vi "State Exit.vi"(8 "error in":errorcluster, 11 "Context in":refnum<class "State Pattern.lvclass">) -> (0 "error out":errorcluster, 3 "Context out":refnum<class "State Pattern.lvclass">)   [LabVIEW 2021, in "State Pattern.lvclass"]
uses:
  State Pattern.lvclass
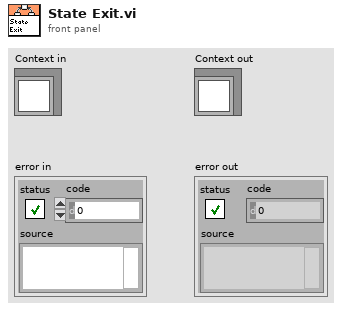
[diagram p1: front panel]
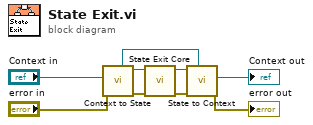
[diagram p0: block diagram]
diagram:
  n1 = call "Context to State.vi"("error in"="error in", "Context in"="Context in") -> ("error out"=w8:errorcluster, "State out"=w3:refnum<class "State Pattern.lvclass">, "Context out (for Preserve Run-Time Class)"=w6:refnum<class "State Pattern.lvclass">)  [unwired: 7 in]
  n2 = call-dynamic "State Exit Core.vi"("error in"=w8, "State in"=w3) -> ("error out"=w7:errorcluster, "State out"=w2:refnum<class "State Pattern.lvclass">)  [unwired: 8 in]
  n3 = call "State to Context.vi"("Context in (for Preserve Run-Time Class)"=w6, "error in"=w7, "State in"=w2) -> ("error out"=→"error out":errorcluster, "Context out"=→"Context out":refnum<class "State Pattern.lvclass">)  [unwired: 7 in]
